vi "DVW_Size Waveform.vi"(3 "DVW":T1) -> (1 "Size Out":i32)   [LabVIEW 2015]
uses:
  TypeDefs_Utility/Ref_DVR_Buffer.ctl
  Universal Controls/Waveform_Data.ctl
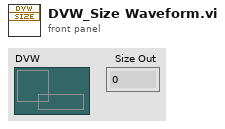
[diagram p1: front panel]
types:
  T1 = typedef "Ref_DVR_Buffer.ctl" = refnum<data-value>
  T2 = typedef "Waveform_Data.ctl" = waveform(dbl)
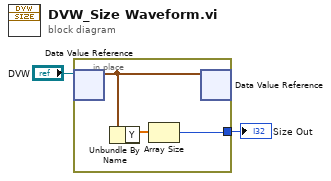
[diagram p0: block diagram]
diagram:
  n1 = in-place {
    in-place-border: [w3] -> w1
    n2 = in-place-dvr #1("DVW") -> (w5:T2)  [unwired: 1 out]
    n3 = Unbundle By Name(w5) -> ("Y"=w4:dbl[])
    n4 = Array Size(array=w4) -> (size(s)=w3:i32)
    n5 = in-place-dvr #1(w5) -> ()  [unwired: 2 out]
  }
  "Size Out" <- w1
